vi "Calibrate_Sums.vi"(8 "error in (no error)":errorcluster, 11 "Signal Channel":enum16{"Red", "Green"}(ring)) -> (0 "error out":errorcluster, 2 "Y Distance Array":sgl[](array[numeric]), 3 "X Distance Array":sgl[](array[numeric]))   [LabVIEW 2020]
doc: "Use this template to create a dialog box with event handling."
uses:
  Typedefs/Top level VI states.ctl
  TypeDefs/Control Plane.ctl
  Globals/gl_Calibration globals.vi
  Global Variables/gl_Images.vi
  Global Variables/General Globals.vi
panel:
  in  "Delay 3":u32=1000
  out "Image 2":T1(plugin-control)
  out "Image":T1(plugin-control)
  in  "Delay 2":u32=1000
  in  "Delay":u32=1000
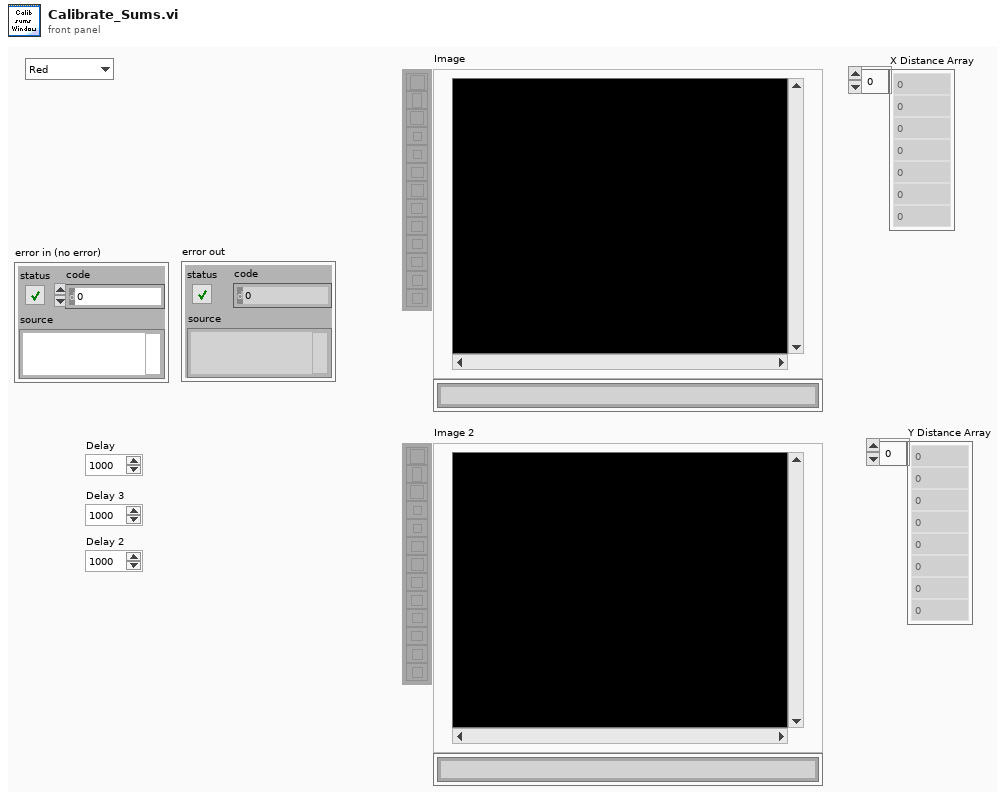
[diagram p1: front panel]
types:
  T1 = typedef "IMAQ Image.ctl" = refnum<image>
  T2 = enum16{"Raster", "Structural", "Pointing", "Mini Scan", "Alignment"}
  T3 = typedef "Top level VI states.ctl" = enum16{"None", "Initialise UI", "<STACK PROTOCOL STATES>", "AOL Zstack-START", "AOL Zstack-STOP", "Motor Zstack-START", "Motor Zstack-STOP", "<ACQUISITION PROTOCOL STATES> ", "Functional Acquisition-START", "Functional Acquisition-STOP", "Single Plane Acquisition-START", "Single Plane Acquisition-STOP", "Volume Acquisition-START", "Volume Acquisition-STOP", "<LIVE IMAGING PROTOCOL STATES>", "Live Imaging-START", "Live Imaging-STOP", "Live Plane Imaging-START", "Live Plane Imaging-STOP", "Live Volume Imaging-START", "Live Volume Imaging-STOP", "<MOVEMENT CORRECTION PROTOCOL STATES>", "EXIT"}
  T4 = typedef "Control Plane.ctl" = enum16{"XY-X", "XY-Y", "Z"}
  T5 = typedef "General Scan Parameters.ctl" = cluster{"Field of View":sgl, "Frame Size":u16, "Dwell Time (ms)":dbl, "Wavelength (nm)":dbl, "Zoom":dbl, "AOL Xc":sgl, "AOL Yc":sgl, "AOL Zc":sgl, "AOL Mode":enum16{"Raster", "Structural", "Pointing", "Mini Scan", "Alignment"}, "Imaging Mode":enum16{"Live Imaging", "AOL Zstack", "Motor Zstack", "Functional Imaging"}}
  T6 = typedef "Current Calibration Parameters.ctl" = cluster{"Sum X":dbl, "Sum Y":dbl, "Diff X":dbl, "Diff Y":dbl, "Distortion Correction":dbl, "Z_norm to um_scaling":dbl, "X_norm to um_scaling":dbl, "Samples to Wait after Trigger":dbl, "Slip Cycle":dbl}
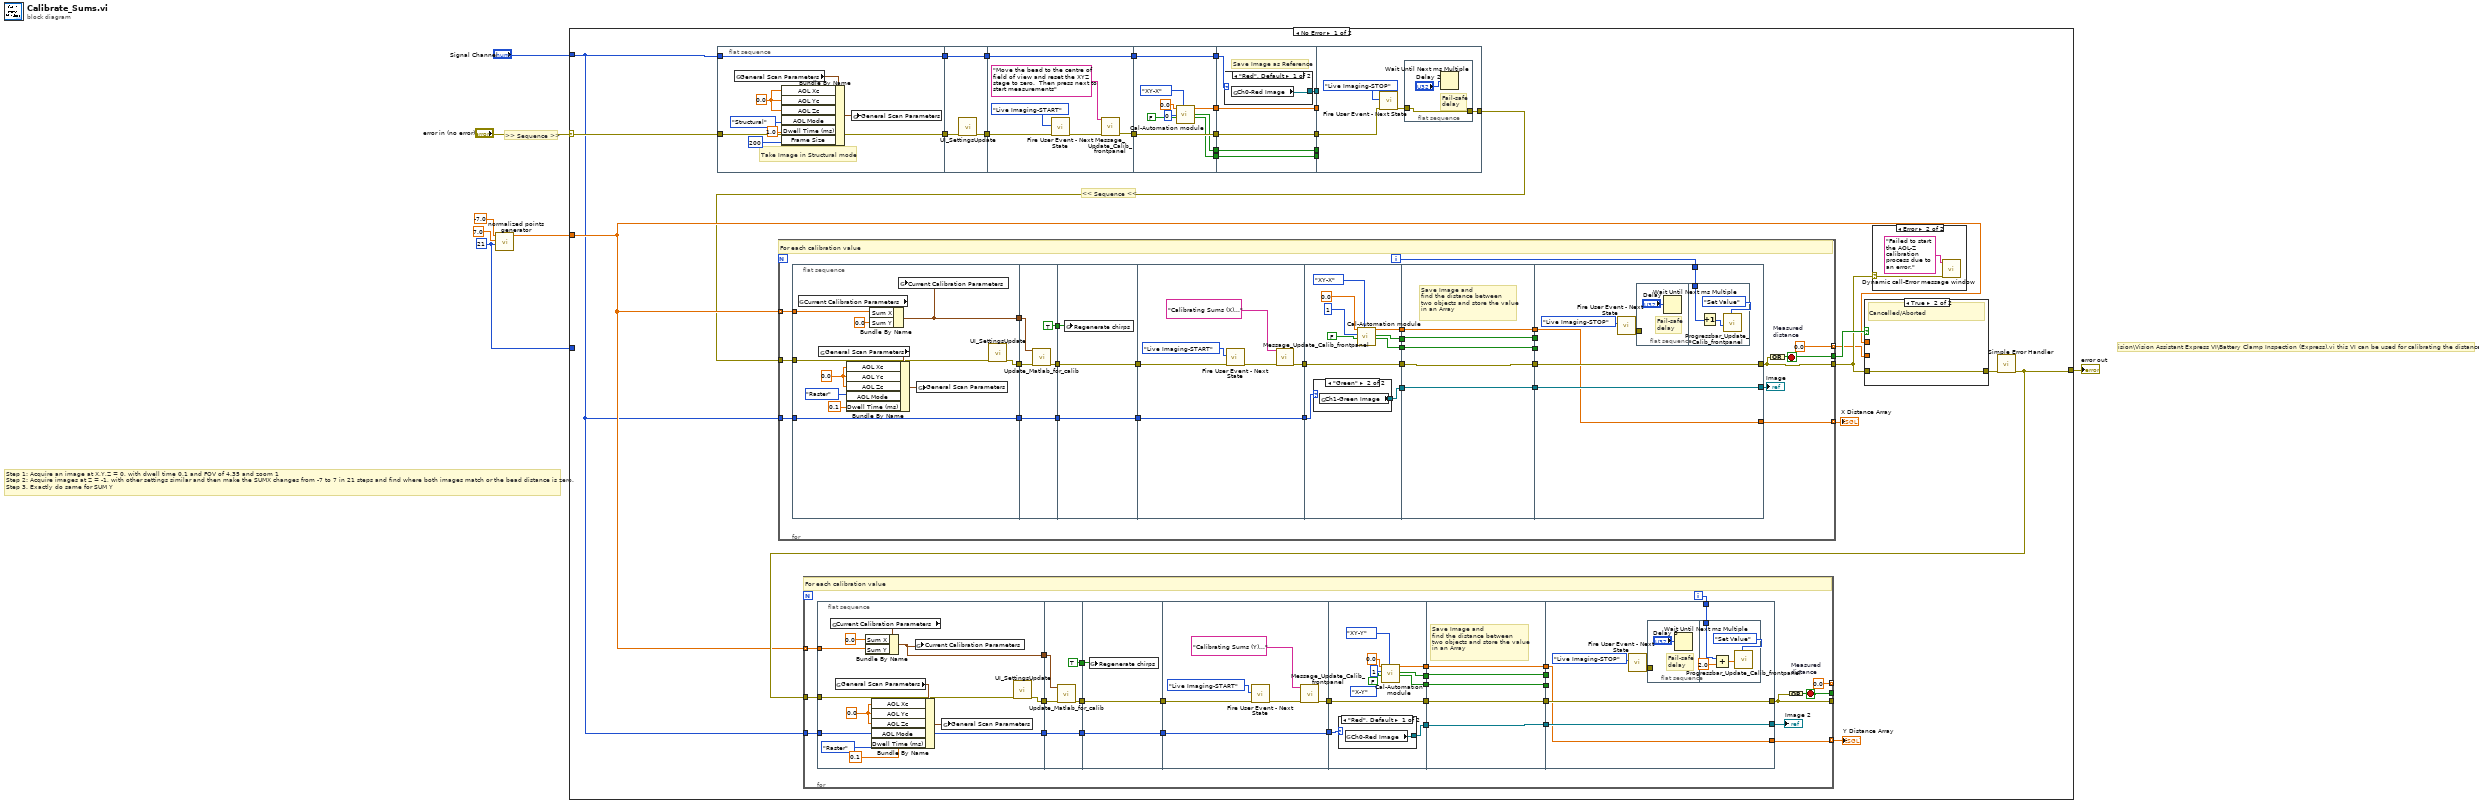
[diagram p0: block diagram]
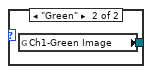
[diagram p2: hidden frame]
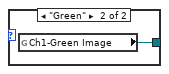
[diagram p3: hidden frame]
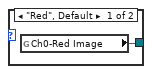
[diagram p4: hidden frame]
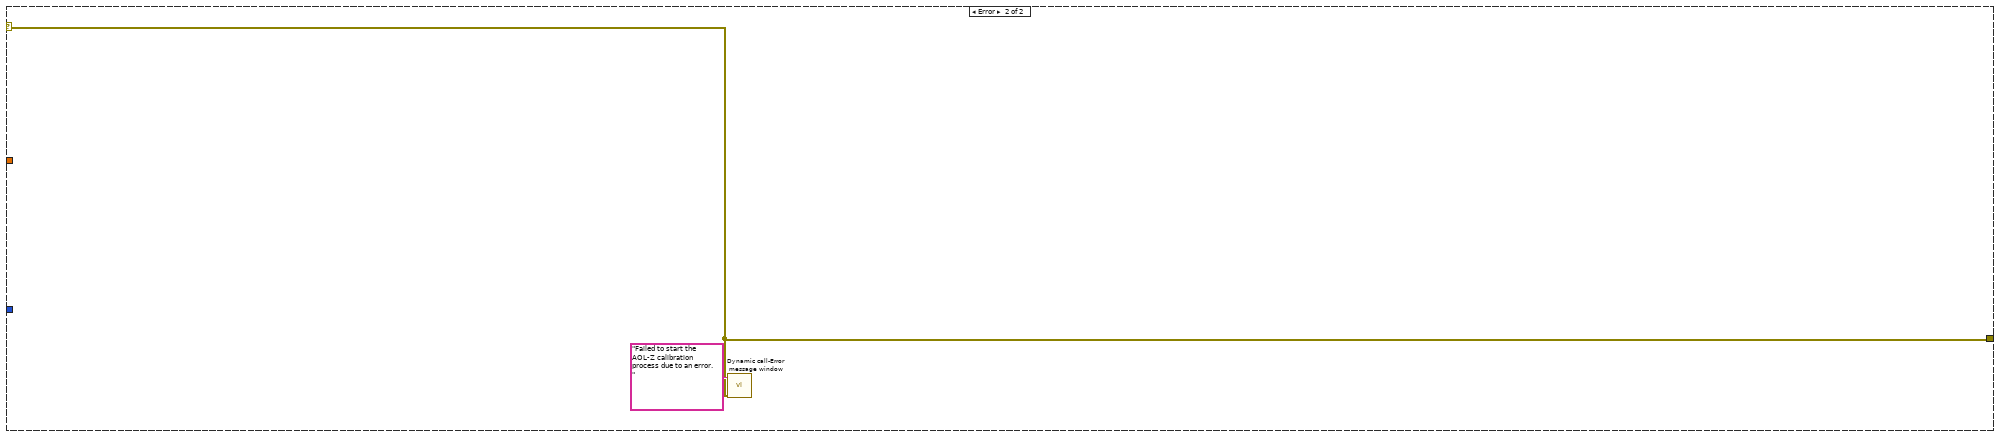
[diagram p7: hidden frame]
diagram:
  w1 = 21 ("number of points")
  # ">> Sequence >>"
  # "ision\\Vision Assistant Express VI\\Battery Clamp Inspection (Express).vi this VI can be used for calibrating the distance"
  # "Step 1: Acquire an image at X,Y,Z = 0, with dwell time 0.1 and FOV of 4.35 and zoom 1\nStep 2: Acquire images at Z = -1, with other settings similar and then make the SUMX changes from -7 to 7 in 21 steps and find where both images match or the bead distance is zero.\nStep 3. Exactly do same for SUM Y"
  n1 = call "normalized points generator.vi"("number of points"=w1, "maximum"=7.0, "minimum"=-7.0) -> ("normalised array"=w5:dbl[])  [unwired: 7 in, 1 out]
  n2 = case shown="No Error" "error in (no error)" {
    selector: "error in (no error)" -> [w28 w243]
    tunnel: w5 -> [w12 _]
    tunnel: [w13 w243] -> w7
    tunnel: "Signal Channel" -> [w10 _]
    tunnel: w1 -> [_ _]
    frame No Error {
      # "<< Sequence <<"
      n3 = flat-sequence {
        tunnel: w28 -> [w122]
        tunnel: [w122] -> w29
        tunnel: [w121] -> w15
        tunnel: w10 -> [w121]
        tunnel: [w128] -> w31
        tunnel: w29 -> [w127]
        tunnel: [w126] -> w16
        tunnel: w15 -> [w126]
        tunnel: [w133] -> w30
        tunnel: w31 -> [w134]
        tunnel: [w129] -> w17
        tunnel: w16 -> [w129]
        tunnel: [w142] -> w20
        tunnel: [w143] -> w22
        tunnel: w30 -> [w143]
        tunnel: [w138] -> w24
        tunnel: [w139] -> w26
        tunnel: [w136] -> w18
        tunnel: w17 -> [w136]
        tunnel: w26 -> [w149]
        tunnel: [w149] -> w25
        tunnel: w24 -> [w148]
        tunnel: [w148] -> w23
        tunnel: w22 -> [w147]
        tunnel: [w147] -> w21
        tunnel: w20 -> [w144]
        tunnel: [w144] -> w19
        tunnel: w18 -> [w146]
        tunnel: [w145] -> w14
        tunnel: w25 -> [_]
        tunnel: w23 -> [_]
        tunnel: w21 -> [w153]
        tunnel: w19 -> [_]
        tunnel: w14 -> [_]
        tunnel: [w152] -> w11
        frame #0 {
          w123 = sgl 0.0 ("AOL Yc")
          # "Take Image in Structural mode"
          n4 = global read "gl_Calibration globals.vi" "General Scan Parameters"() -> (w125:T5)
          n5 = Bundle By Name(cluster=w125, "AOL Xc"=w123, "AOL Yc"=w123, "AOL Zc"=w123, "AOL Mode"=T2."Structural", "Dwell Time (ms)"=1.0, "Frame Size"=u16 200) -> (w124:T5)
          n6 = global write "gl_Calibration globals.vi" "General Scan Parameters"(w124) -> ()
        }
        frame #1 {
          n7 = call "UI_SettingsUpdate.vi"("error in (no error)"=w127) -> ("error out"=w128:errorcluster)  [unwired: 10 in]
        }
        frame #2 {
          n8 = call "Fire User Event - Next State.vi"("Error In"=w134, "\"UI Handler loop\" case to execute"=Top_level_VI_states."Live Imaging-START" ("\"UI Handler loop\" case to execute")) -> ("Error Out"=w132:errorcluster)  [unwired: 9 in]
          n9 = call "Message_Update_Calib_frontpanel.vi"("error in (no error)"=w132, "Message"="Move the bead to the centre of field of view and reset the XYZ stage to zero.  Then press next to start measurements") -> ("error out"=w133:errorcluster)  [unwired: 9 in]
        }
        frame #3 {
          n10 = call "Cal-Automation module.vi"("Parameter"=Control_Plane."XY-X", "Timed out while waiting for acknowledgement in"=FALSE, "FOR loop index"=0, "Initial motor position (um)"=sgl 0.0) -> ("Motor timed out or errored out"=w138:bool, "Cancelled"=w139:bool, "Measured cal value"=w142:sgl)  [unwired: 4 in, 1 out]
        }
        frame #4 {
          # "Save Image as Reference"
          n11 = case shown="\"Red\", Default" w146 {
            tunnel: [w150 w151] -> w145
            frame "Red", Default {
              n12 = global read "gl_Images.vi" "Ch0-Red Image"() -> (w150:T1)
            }
            frame "Green" {
              n13 = global read "gl_Images.vi" "Ch1-Green Image"() -> (w151:T1)
            }
          }
        }
        frame #5 {
          n14 = call "Fire User Event - Next State.vi"("Error In"=w153, "\"UI Handler loop\" case to execute"=Top_level_VI_states."Live Imaging-STOP" ("\"UI Handler loop\" case to execute")) -> ("Error Out"=w155:errorcluster)  [unwired: 9 in]
          n15 = flat-sequence {
            tunnel: w155 -> [w156]
            tunnel: [w156] -> w152
            frame #0 {
              # "Fail-safe delay"
              n16 = Wait Until Next ms Multiple(millisecond multiple="Delay 2") -> ()  [unwired: 1 out]
            }
          }
        }
      }
      n17 = for {
        tunnel: w12 -> [w186] mode=indexing
        tunnel: [w181] -> w33
        tunnel: [w182] -> w32
        tunnel: w11 -> [w184]
        tunnel: [w172] -> w27 mode=indexing
        tunnel: w10 -> [w171]
        tunnel: [w158] -> w9 mode=indexing
        i -> [w161]
        stop <- w181 stop-if-true
        w172 = sgl 0.0  # Measured  distance
        # "For each calibration value"
        n18 = flat-sequence {
          tunnel: w186 -> [w197]
          tunnel: w184 -> [w188]
          tunnel: [w187] -> w183
          tunnel: [w196] -> w173
          tunnel: w171 -> [w194]
          tunnel: [w194] -> w170
          tunnel: w183 -> [w203]
          tunnel: [w202] -> w167
          tunnel: w173 -> [w201]
          tunnel: w170 -> [w200]
          tunnel: [w200] -> w165
          tunnel: [TRUE] -> w163
          tunnel: w167 -> [w206]
          tunnel: [w206] -> w166
          tunnel: w165 -> [w205]
          tunnel: [w205] -> w164
          tunnel: w163 -> [w204]
          tunnel: [w211] -> w185
          tunnel: w166 -> [w212]
          tunnel: w164 -> [w207]
          tunnel: [w207] -> w169
          tunnel: [w221] -> w180
          tunnel: [w222] -> w179
          tunnel: w185 -> [w222]
          tunnel: [w217] -> w177
          tunnel: [w218] -> w175
          tunnel: w169 -> [w214]
          tunnel: [w215] -> w168
          tunnel: w180 -> [w225]
          tunnel: w179 -> [w227]
          tunnel: [w227] -> w178
          tunnel: w177 -> [w229]
          tunnel: [w229] -> w176
          tunnel: w175 -> [w228]
          tunnel: [w228] -> w174
          tunnel: w168 -> [w226]
          tunnel: [w226] -> w160
          tunnel: [w225] -> w159
          tunnel: w178 -> [w234]
          tunnel: [w234] -> w182
          tunnel: w176 -> [_]
          tunnel: w174 -> [_]
          tunnel: [w232] -> w162
          tunnel: w161 -> [w231]
          tunnel: w160 -> [w232]
          tunnel: w159 -> [w230]
          tunnel: [w230] -> w158
          frame #0 {
            w191 = sgl 0.0 ("AOL Yc")
            n19 = global read "gl_Calibration globals.vi" "Current Calibration Parameters"() -> (w198:T6)
            n20 = global read "gl_Calibration globals.vi" "General Scan Parameters"() -> (w193:T5)
            n21 = Bundle By Name(cluster=w193, "AOL Xc"=w191, "AOL Yc"=w191, "AOL Zc"=w191, "AOL Mode"=T2."Raster", "Dwell Time (ms)"=0.1) -> (w192:T5)
            n22 = Bundle By Name(cluster=w198, "Sum X"=w197, "Sum Y"=0.0) -> (w196:T6)
            n23 = global write "gl_Calibration globals.vi" "Current Calibration Parameters"(w196) -> ()
            n24 = global write "gl_Calibration globals.vi" "General Scan Parameters"(w192) -> ()
            n25 = call "UI_SettingsUpdate.vi"("error in (no error)"=w188) -> ("error out"=w187:errorcluster)  [unwired: 10 in]
          }
          frame #1 {
            n26 = call "Update_Matlab_for_calib.vi"("error in (no error)"=w203, "Current Calibration Parameters"=w201) -> ("error out"=w202:errorcluster)  [unwired: 9 in]
          }
          frame #2 {
            n27 = global write "General Globals.vi" "Regenerate chirps"(w204) -> ()
          }
          frame #3 {
            n28 = call "Fire User Event - Next State.vi"("Error In"=w212, "\"UI Handler loop\" case to execute"=Top_level_VI_states."Live Imaging-START" ("\"UI Handler loop\" case to execute")) -> ("Error Out"=w210:errorcluster)  [unwired: 9 in]
            n29 = call "Message_Update_Calib_frontpanel.vi"("error in (no error)"=w210, "Message"="Calibrating Sums (X)...") -> ("error out"=w211:errorcluster)  [unwired: 9 in]
          }
          frame #4 {
            n30 = case shown="\"Green\"" w214 {
              tunnel: [w223 w224] -> w215
              frame "Red", Default {
                n31 = global read "gl_Images.vi" "Ch0-Red Image"() -> (w223:T1)
              }
              frame "Green" {
                n32 = global read "gl_Images.vi" "Ch1-Green Image"() -> (w224:T1)
              }
            }
            n33 = call "Cal-Automation module.vi"("Parameter"=Control_Plane."XY-X", "Timed out while waiting for acknowledgement in"=FALSE, "FOR loop index"=1, "Initial motor position (um)"=sgl 0.0) -> ("Motor timed out or errored out"=w217:bool, "Cancelled"=w218:bool, "Measured cal value"=w221:sgl)  [unwired: 4 in, 1 out]
          }
          frame #5 {
            # "Save Image and \nfind the distance between\ntwo objects and store the value\nin an Array"
          }
          frame #6 {
            n34 = call "Fire User Event - Next State.vi"("\"UI Handler loop\" case to execute"=Top_level_VI_states."Live Imaging-STOP" ("\"UI Handler loop\" case to execute")) -> ("Error Out"=w235:errorcluster)  [unwired: 10 in]
            n35 = flat-sequence {
              tunnel: w235 -> [_]
              tunnel: w231 -> [w238]
              frame #0 {
                # "Fail-safe delay"
                n36 = Wait Until Next ms Multiple(millisecond multiple="Delay") -> ()  [unwired: 1 out]
              }
              frame #1 {
                n37 = Increment(x=w238) -> (x+1=w237:i32)
                n38 = call "Progressbar_Update_Calib_frontpanel.vi"("Ops"=enum16{"Set Value", "Set Range"}."Set Value", "Value"=w237) -> ()  [unwired: 9 in, 1 out]
              }
            }
          }
        }
        n39 = Compound Arithmetic op=OR(w182) -> (w181:bool)
        "Image" <- w162
      }
      "X Distance Array" <- w9
      n40 = case shown="True" w33 {
        tunnel: w12 -> [_ _]
        tunnel: w27 -> [_ _]
        tunnel: [_ w242] -> w34
        tunnel: w32 -> [_ w242]
        frame False {
          # "find zero value from the array"
        }
        frame True {
          # "Cancelled/Aborted"
        }
      }
      n41 = case shown="Error" w32 {
        selector: w32 -> [_ w241]
        frame No Error {
        }
        frame Error {
          n42 = call "Dynamic call-Error message window.vi"("error in (no error)"=w241, "Error Message"="Failed to start the AOL-Z calibration process due to an error.") -> ()  [unwired: 9 in, 1 out]
        }
      }
      n43 = call <vilib>:"Simple Error Handler.vi"("error in (no error)"=w34) -> ("error out"=w13:errorcluster)  [unwired: 4 in, 4 out]
      n44 = for {
        tunnel: w12 -> [w63] mode=indexing
        tunnel: [w58] -> _
        tunnel: [w59] -> _
        tunnel: w13 -> [w61]
        tunnel: [w49] -> _ mode=indexing
        tunnel: w10 -> [w48]
        tunnel: [w35] -> w8 mode=indexing
        i -> [w37]
        stop <- w58 stop-if-true
        w49 = sgl 0.0  # Measured  distance
        # "For each calibration value"
        n45 = flat-sequence {
          tunnel: w63 -> [w64]
          tunnel: w61 -> [w67]
          tunnel: [w66] -> w60
          tunnel: [w74] -> w50
          tunnel: w48 -> [w73]
          tunnel: [w73] -> w47
          tunnel: w60 -> [w80]
          tunnel: [w79] -> w44
          tunnel: w50 -> [w78]
          tunnel: w47 -> [w77]
          tunnel: [w77] -> w42
          tunnel: [TRUE] -> w40
          tunnel: w44 -> [w83]
          tunnel: [w83] -> w43
          tunnel: w42 -> [w82]
          tunnel: [w82] -> w41
          tunnel: w40 -> [w81]
          tunnel: [w88] -> w62
          tunnel: w43 -> [w89]
          tunnel: w41 -> [w84]
          tunnel: [w84] -> w46
          tunnel: [w98] -> w57
          tunnel: [w99] -> w56
          tunnel: w62 -> [w99]
          tunnel: [w94] -> w54
          tunnel: [w95] -> w52
          tunnel: w46 -> [w91]
          tunnel: [w92] -> w45
          tunnel: w57 -> [w102]
          tunnel: w56 -> [w104]
          tunnel: [w104] -> w55
          tunnel: w54 -> [w106]
          tunnel: [w106] -> w53
          tunnel: w52 -> [w105]
          tunnel: [w105] -> w51
          tunnel: w45 -> [w103]
          tunnel: [w103] -> w39
          tunnel: [w102] -> w36
          tunnel: w55 -> [w111]
          tunnel: [w111] -> w59
          tunnel: w53 -> [_]
          tunnel: w51 -> [_]
          tunnel: [w109] -> w38
          tunnel: w39 -> [w109]
          tunnel: w37 -> [w108]
          tunnel: w36 -> [w107]
          tunnel: [w107] -> w35
          frame #0 {
            w70 = sgl 0.0 ("AOL Yc")
            n46 = global read "gl_Calibration globals.vi" "Current Calibration Parameters"() -> (w75:T6)
            n47 = global read "gl_Calibration globals.vi" "General Scan Parameters"() -> (w72:T5)
            n48 = Bundle By Name(cluster=w75, "Sum X"=0.0 ("Sum Y"), "Sum Y"=w64) -> (w74:T6)
            n49 = Bundle By Name(cluster=w72, "AOL Xc"=w70, "AOL Yc"=w70, "AOL Zc"=w70, "AOL Mode"=T2."Raster", "Dwell Time (ms)"=0.1) -> (w71:T5)
            n50 = global write "gl_Calibration globals.vi" "Current Calibration Parameters"(w74) -> ()
            n51 = global write "gl_Calibration globals.vi" "General Scan Parameters"(w71) -> ()
            n52 = call "UI_SettingsUpdate.vi"("error in (no error)"=w67) -> ("error out"=w66:errorcluster)  [unwired: 10 in]
          }
          frame #1 {
            n53 = call "Update_Matlab_for_calib.vi"("error in (no error)"=w80, "Current Calibration Parameters"=w78) -> ("error out"=w79:errorcluster)  [unwired: 9 in]
          }
          frame #2 {
            n54 = global write "General Globals.vi" "Regenerate chirps"(w81) -> ()
          }
          frame #3 {
            n55 = call "Fire User Event - Next State.vi"("Error In"=w89, "\"UI Handler loop\" case to execute"=Top_level_VI_states."Live Imaging-START" ("\"UI Handler loop\" case to execute")) -> ("Error Out"=w87:errorcluster)  [unwired: 9 in]
            n56 = call "Message_Update_Calib_frontpanel.vi"("error in (no error)"=w87, "Message"="Calibrating Sums (Y)...") -> ("error out"=w88:errorcluster)  [unwired: 9 in]
          }
          frame #4 {
            (unwired) enum16{"X-Y", "Z"}."X-Y" ("StageSelection")
            n57 = case shown="\"Red\", Default" w91 {
              tunnel: [w100 w101] -> w92
              frame "Red", Default {
                n58 = global read "gl_Images.vi" "Ch0-Red Image"() -> (w100:T1)
              }
              frame "Green" {
                n59 = global read "gl_Images.vi" "Ch1-Green Image"() -> (w101:T1)
              }
            }
            n60 = call "Cal-Automation module.vi"("Parameter"=Control_Plane."XY-Y", "Timed out while waiting for acknowledgement in"=FALSE, "FOR loop index"=1, "Initial motor position (um)"=sgl 0.0) -> ("Motor timed out or errored out"=w94:bool, "Cancelled"=w95:bool, "Measured cal value"=w98:sgl)  [unwired: 4 in, 1 out]
          }
          frame #5 {
            # "Save Image and \nfind the distance between\ntwo objects and store the value\nin an Array"
          }
          frame #6 {
            n61 = call "Fire User Event - Next State.vi"("\"UI Handler loop\" case to execute"=Top_level_VI_states."Live Imaging-STOP" ("\"UI Handler loop\" case to execute")) -> ("Error Out"=w112:errorcluster)  [unwired: 10 in]
            n62 = flat-sequence {
              tunnel: w112 -> [_]
              tunnel: w108 -> [w114]
              frame #0 {
                # "Fail-safe delay"
                n63 = Wait Until Next ms Multiple(millisecond multiple="Delay 3") -> ()  [unwired: 1 out]
              }
              frame #1 {
                n64 = Add(x=w114, y=2.0) -> (x+y=w115:dbl)
                n65 = call "Progressbar_Update_Calib_frontpanel.vi"("Ops"=enum16{"Set Value", "Set Range"}."Set Value", "Value"=w115) -> ()  [unwired: 9 in, 1 out]
              }
            }
          }
        }
        n66 = Compound Arithmetic op=OR(w59) -> (w58:bool)
        "Image 2" <- w38
      }
      "Y Distance Array" <- w8
    }
    frame Error {
      n67 = call "Dynamic call-Error message window.vi"("error in (no error)"=w243, "Error Message"="Failed to start the AOL-Z calibration process due to an error.") -> ()  [unwired: 9 in, 1 out]
    }
  }
  "error out" <- w7
